vi "Gradient Example.vi"() -> ()   [LabVIEW 2012]
uses:
  User Controls/Array Dimensions.ctl
  Non-User VIs/Allocate Memory/AllocateMemory_32f.vi
  Non-User VIs/Functions/Gradient/Create Gradient 32f.vi
  Non-User VIs/Functions/Gradient/Delete Gradient 32f.vi
  Non-User VIs/Error Checking/View Error Log Mode Functional Global.vi
  Non-User VIs/Write Memory/WriteMemory_32f.vi
  Non-User VIs/Functions/Gradient/Compute Gradient 32f.vi
  Non-User VIs/Read Memory/ReadMemory_32f.vi
  OpenCLV x64.lvlib
panel:
  out "Z":sgl[][][](array[numeric])
  out "Y":sgl[][][](array[numeric])
  out "X":sgl[][][](array[numeric])
  out "Time in ms":u32=149
  in  "Dimension":T1={"Depth"=97, "Height"=512, "Width"=191} {"Width" min=1; "Height" min=1; "Depth" min=1}
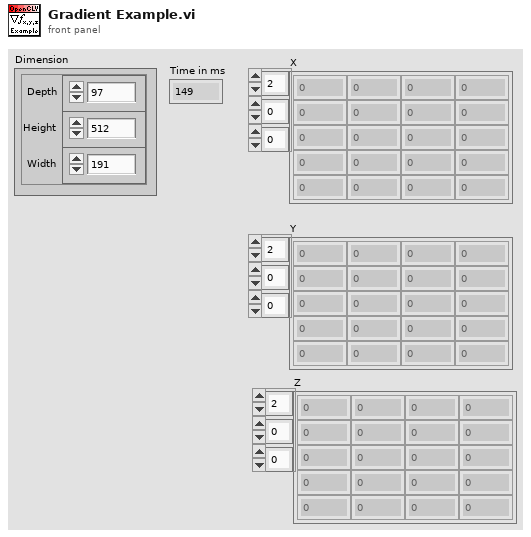
[diagram p1: front panel]
types:
  T1 = typedef "Array Dimensions.ctl" = cluster{"Depth":u64, "Height":u64, "Width":u64}
  T2 = typedef "OpenCLV x64.lvlib/Device ID.ctl" = u64
  T3 = typedef "OpenCLV x64.lvlib/Memory Object.ctl" = cluster{"Device ID":T2, "Memeroy ID":T4, "Dimension":T1, "Memory Type":T5}
  T4 = typedef "OpenCLV x64.lvlib/Memory ID.ctl" = u64
  T5 = typedef "OpenCLV x64.lvlib/Memory Type.ctl" = enum16{"32f", "u8", "i8", "u16", "i16", "u32", "i32", "64f"}
  T6 = typedef "OpenCLV x64.lvlib/Gradient Object.ctl" = cluster{"Program Handle":T7, "Device Out":T2, "X":T3, "Y":T3, "Z":T3}
  T7 = typedef "OpenCLV x64.lvlib/Program Handle.ctl" = u64
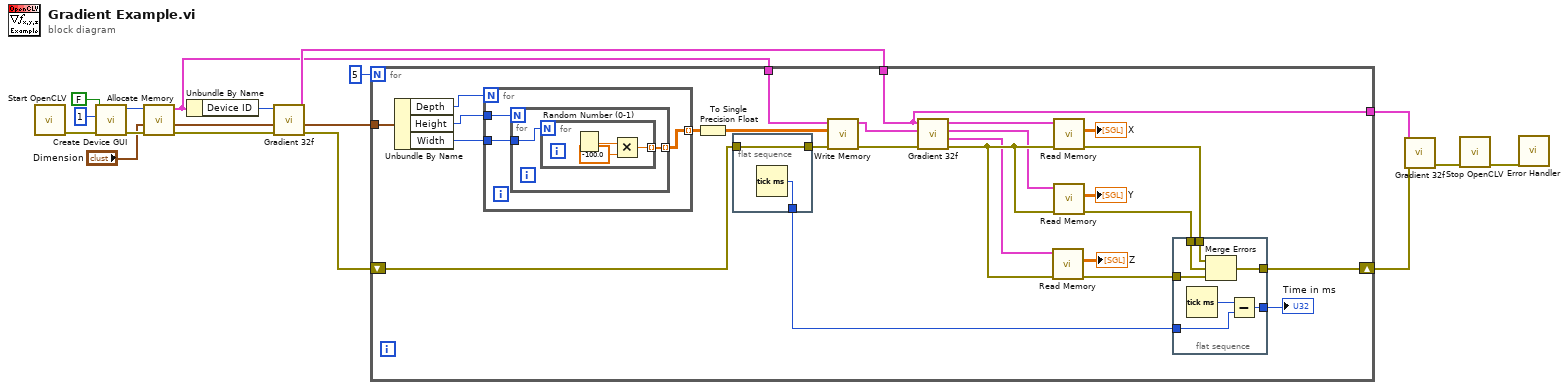
[diagram p0: block diagram]
diagram:
  n1 = call "Start OpenCLV.vi"() -> ("Error Out"=w18:errorcluster)  [unwired: 11 in]
  n2 = call "Create Device GUI.vi"("Error In"=w18, "Platform"=1, "Skip Configuration"=FALSE) -> ("error constant"=w17:errorcluster, "Device Reference"=w16:T2)  [unwired: 7 in]
  n3 = call-poly "Allocate Memory.vi"("Error In"=w17, "Dimension"="Dimension", "Device In"=w16) -> ("Error Out"=w9:errorcluster, "Dimension Out"=w5:T1, "Memory Object"=w3:T3)  [unwired: 6 in]
  n4 = Unbundle By Name(w3) -> ("Device ID"=w6:T2)
  n5 = call-poly "Gradient 32f.vi"("Error In"=w9, "Dimension"=w5, "Device In"=w6) -> ("Error Out"=w8:errorcluster, "Dimension Out"=w4:T1, "Gradient Object"=w7:T6)  [unwired: 6 in]
  n6 = for {
    N: 5 -> [_]
    tunnel: [w39] -> w13
    tunnel: w7 -> [w39]
    tunnel: w4 -> [w37]
    tunnel: w3 -> [w36]
    shift-right: [w40] -> w14
    shift-left: w8 -> [w22]
    n7 = Unbundle By Name(w37) -> ("Depth"=w43:u64, "Height"=w42:u64, "Width"=w41:u64)
    n8 = for {
      N: w43 -> [_]
      tunnel: w42 -> [w55]
      tunnel: w41 -> [w54]
      tunnel: [w53] -> w38 mode=indexing
      n9 = for {
        N: w55 -> [_]
        tunnel: w54 -> [w57]
        tunnel: [w56] -> w53 mode=indexing
        n10 = for {
          N: w57 -> [_]
          tunnel: [w58] -> w56 mode=indexing
          n11 = Random Number (0-1)() -> (number: 0 to 1=w60:dbl)
          n12 = Multiply(x=w60, y=-100.0) -> (x*y=w58:dbl)
        }
      }
    }
    n13 = To Single Precision Float(number=w38) -> (single precision float=w35:sgl[][][])
    n14 = flat-sequence {
      tunnel: w22 -> [w52]
      tunnel: [w52] -> w21
      tunnel: [w51] -> w20
      frame #0 {
        n15 = Tick Count (ms)() -> (millisecond timer value=w51:u32)
      }
    }
    n16 = call-poly "Write Memory.vi"("Error In"=w21, "Data In"=w35, "Memory Object In"=w36) -> ("Error Out"=w24:errorcluster, "Memory Object Out"=w23:T3)  [unwired: 6 in, 1 out]
    n17 = call-poly "Gradient 32f.vi"("Error In"=w24, "Input"=w23, "Gradient Object"=w39) -> ("Error Out"=w34:errorcluster, "Z"=w31:T3, "Y"=w32:T3, "X"=w33:T3)  [unwired: 4 in, 1 out]
    n18 = call-poly "Read Memory.vi"("Error In"=w34, "Memory Object In"=w31) -> ("Error Out"=w30:errorcluster, "Data Out"=→"Z":sgl[][][])  [unwired: 6 in, 2 out]
    n19 = call-poly "Read Memory.vi"("Error In"=w34, "Memory Object In"=w33) -> ("Error Out"=w28:errorcluster, "Data Out"=→"X":sgl[][][])  [unwired: 6 in, 2 out]
    n20 = call-poly "Read Memory.vi"("Error In"=w34, "Memory Object In"=w32) -> ("Error Out"=w29:errorcluster, "Data Out"=→"Y":sgl[][][])  [unwired: 6 in, 2 out]
    n21 = flat-sequence {
      tunnel: [w50] -> w40
      tunnel: w30 -> [w49]
      tunnel: w29 -> [w48]
      tunnel: w28 -> [w47]
      tunnel: w20 -> [w45]
      tunnel: [w44] -> w19
      frame #0 {
        n22 = Tick Count (ms)() -> (millisecond timer value=w46:u32)
        n23 = Merge Errors(w47, w48, w49) -> (w50:errorcluster)
        n24 = Subtract(x=w46, y=w45) -> (x-y=w44:u32)
      }
    }
    "Time in ms" <- w19
  }
  n25 = call-poly "Gradient 32f.vi"("Error In"=w14, "Gradient Object"=w13) -> ("Error Out"=w12:errorcluster)  [unwired: 9 in]
  n26 = call "Stop OpenCLV.vi"("Error In"=w12) -> ("Error Out"=w1:errorcluster)  [unwired: 10 in]
  n27 = call-poly "Error Handler.vi"("Error In"=w1) -> ()  [unwired: 10 in, 1 out]
